vi "AssertVIExecIdle.vi"(0 "VI Reference In":refnum<vi>, 1 "Test Label":string, 3 "Assert Only? (F)":bool, 11 "Error In":errorcluster, 12 "Assert Interval(10 ms)":u32=10, 13 "Timeout(5 sec)":dbl=5.0) -> (4 "VI Reference Out":refnum<vi>, 6 "Asserted Value":T1(ring), 15 "Error Out":errorcluster)   [LabVIEW 2016, in "Drona.lvlib" / "AssertVI.lvlib"]
doc: "Asserts if the VI is in Idle state.\nThe input control name is given as a string , incase of path, use delimiters inbetween the path."
uses:
  AssertVI.lvlib
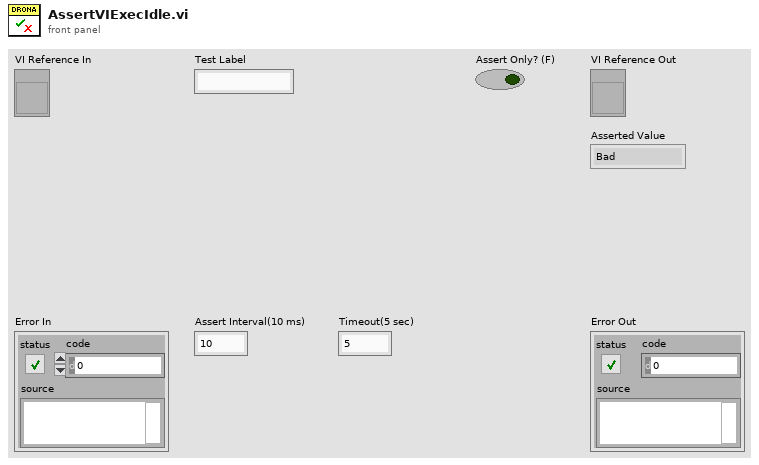
[diagram p1: front panel]
types:
  T1 = enum32{"Bad", "Idle", "Run top level", "Running"}
  T2 = enum32{"Bad", "Idle", "Run top level", "Running"}[]
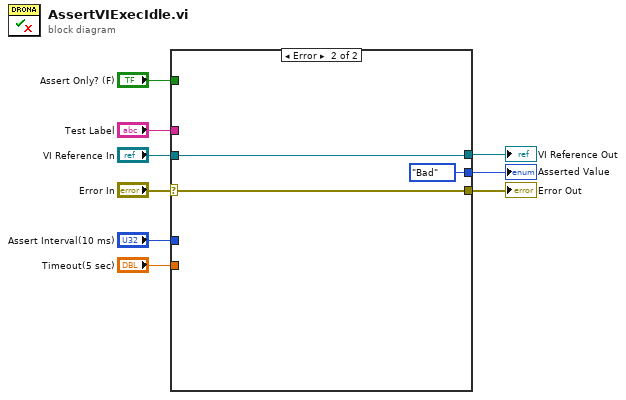
[diagram p0: block diagram]
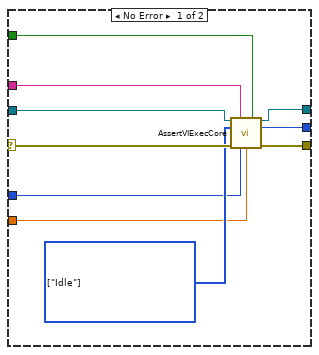
[diagram p2: hidden frame]
diagram:
  n1 = case shown="Error" "Error In" {
    selector: "Error In" -> [w19 w22]
    tunnel: [w18 w22] -> w8
    tunnel: "VI Reference In" -> [w16 w21]
    tunnel: "Test Label" -> [w15 _]
    tunnel: "Assert Only? (F)" -> [w14 _]
    tunnel: "Assert Interval(10 ms)" -> [w13 _]
    tunnel: "Timeout(5 sec)" -> [w12 _]
    tunnel: [w11 w21] -> w2
    tunnel: [w10 T1."Bad" ("Asserted Value")] -> w1
    frame No Error {
      w17 = T2 [enum."Idle"] items=["Bad", "Idle", "Run top level", "Running"] ("Execution:State")
      n2 = call "AssertVIExecCore.vi"("VI Reference In"=w16, "Label"=w15, "Assert Only? (F)"=w14, "Execution:State"=w17, "Error In"=w19, "Assert Interval(10 ms)"=w13, "Timeout(5 sec)"=w12) -> ("VI Reference Out"=w11:refnum<vi>, "Asserted Value"=w10:T1, "Error Out"=w18:errorcluster)  [unwired: 6 in]
    }
    frame Error {
    }
  }
  "Error Out" <- w8
  "VI Reference Out" <- w2
  "Asserted Value" <- w1
